vi "robot movej angle.vi"(0 "robot_id":i32, 7 "参数":T1, 11 "error in (no error)":errorcluster caption="错误输入（无错误）") -> (4 "robot_id out":i32, 6 "function return":i32, 15 "error out":errorcluster caption="错误输出")   [LabVIEW 2020, in "small_scara_interface.lvlib"]
doc: "extern \"C\" __declspec(dllexport) int robot_movej_angle(int robot_id, float angle1, float angle2, float z, float r, float speed, float rough);"
uses:
  small_scara_interface.lvlib
  small_scara_interface.dll
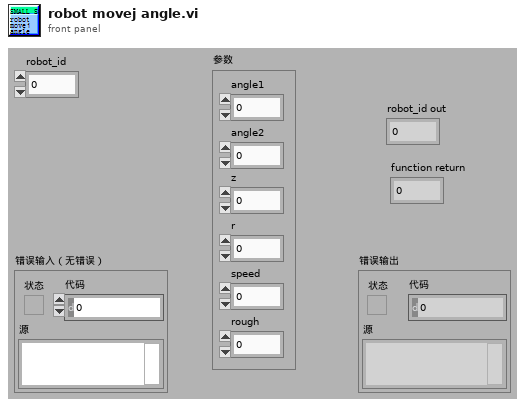
[diagram p1: front panel]
types:
  T1 = cluster{"angle1":sgl, "angle2":sgl, "z":sgl, "r":sgl, "speed":sgl, "rough":sgl}
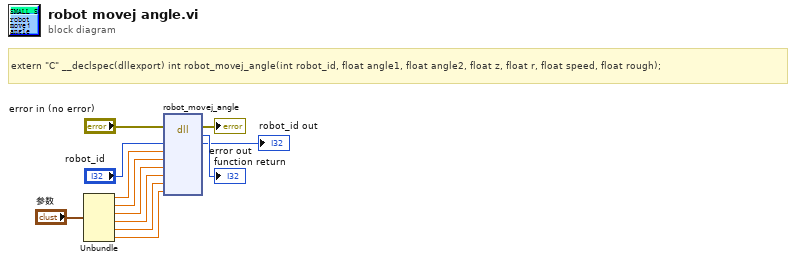
[diagram p0: block diagram]
diagram:
  # "extern \"C\" __declspec(dllexport) int robot_movej_angle(int robot_id, float angle1, float angle2, float z, float r, float speed, float rough);"
  n1 = Unbundle("参数") -> ("angle1"=w6:sgl, "angle2"=w5:sgl, "z"=w4:sgl, "r"=w3:sgl, "speed"=w2:sgl, "rough"=w1:sgl)
  n2 = dll-call lib="PTH2¦abs CUsers\tMogroup-3Desktopé›·èµ›Screening systemlabview multichannel v314subvirobotsubviRobot-HLsmall_scara_interfacesmall_scara_interface.*" fn="robot_movej_angle"(error in="error in (no error)", "robot_id"="robot_id", "angle1"=w6, "angle2"=w5, "z"=w4, "r"=w3, "speed"=w2, "rough"=w1) -> (error out=→"error out":errorcluster, "返回类型"=→"function return":i32, "robot_id"=→"robot_id out":i32)  [unwired: 8 in, 1 out]
